vi "keccak.core.vi"(10 "keccak.i":u16, 11 "state[24]":u64[](array[numeric])=[0, 0, 0, 0, 0, 0, 0, 0, 0, 0, 0, 0, 0, 0, 0, 0, 0, 0, 0, 0, 0, 0, 0, 0] format="%.0x") -> (3 "Ebx":u64[](array[numeric]) format="%.0x")   [LabVIEW 2021]
uses:
  host.impl/Step.4.5.6.7.Inputs.ctl
panel:
  out "New.State":u64[](array[numeric])
  out "Exy":u64[](array[numeric]) format="%.0x"
  out "Step.8.Dx":u64[](array[numeric]) format="%.0x"
  out "state[24].out":u64[](array[numeric]) format="%.0x"
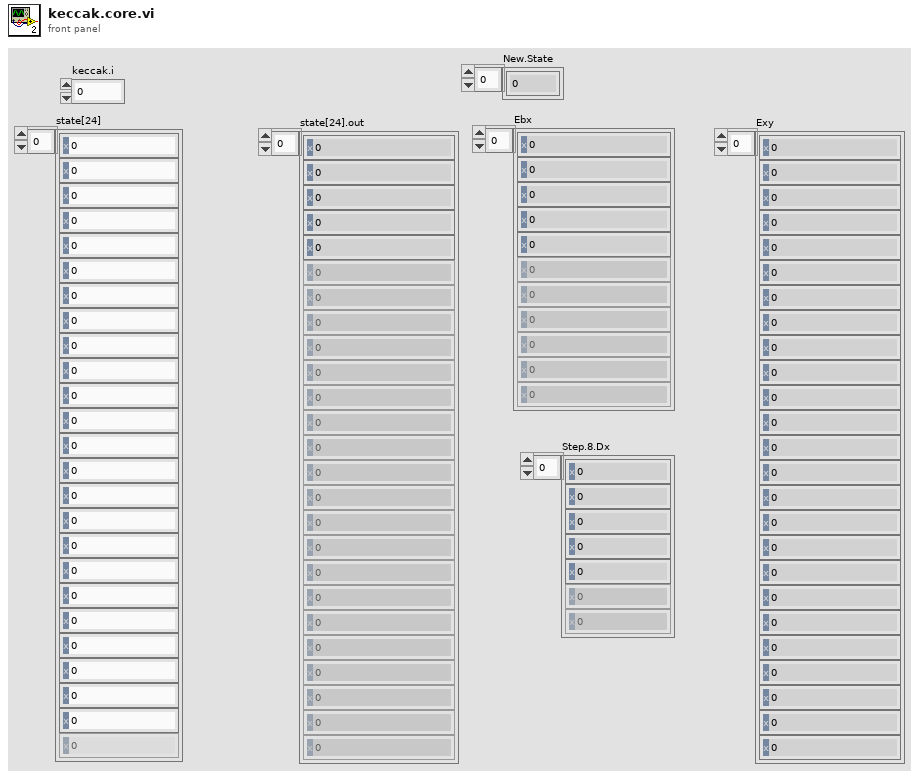
[diagram p1: front panel]
types:
  T1 = typedef "Step.4.5.6.7.Inputs.ctl" = cluster{"Left_Shift":i32, "State_Index":i32, "D_Index":i32}
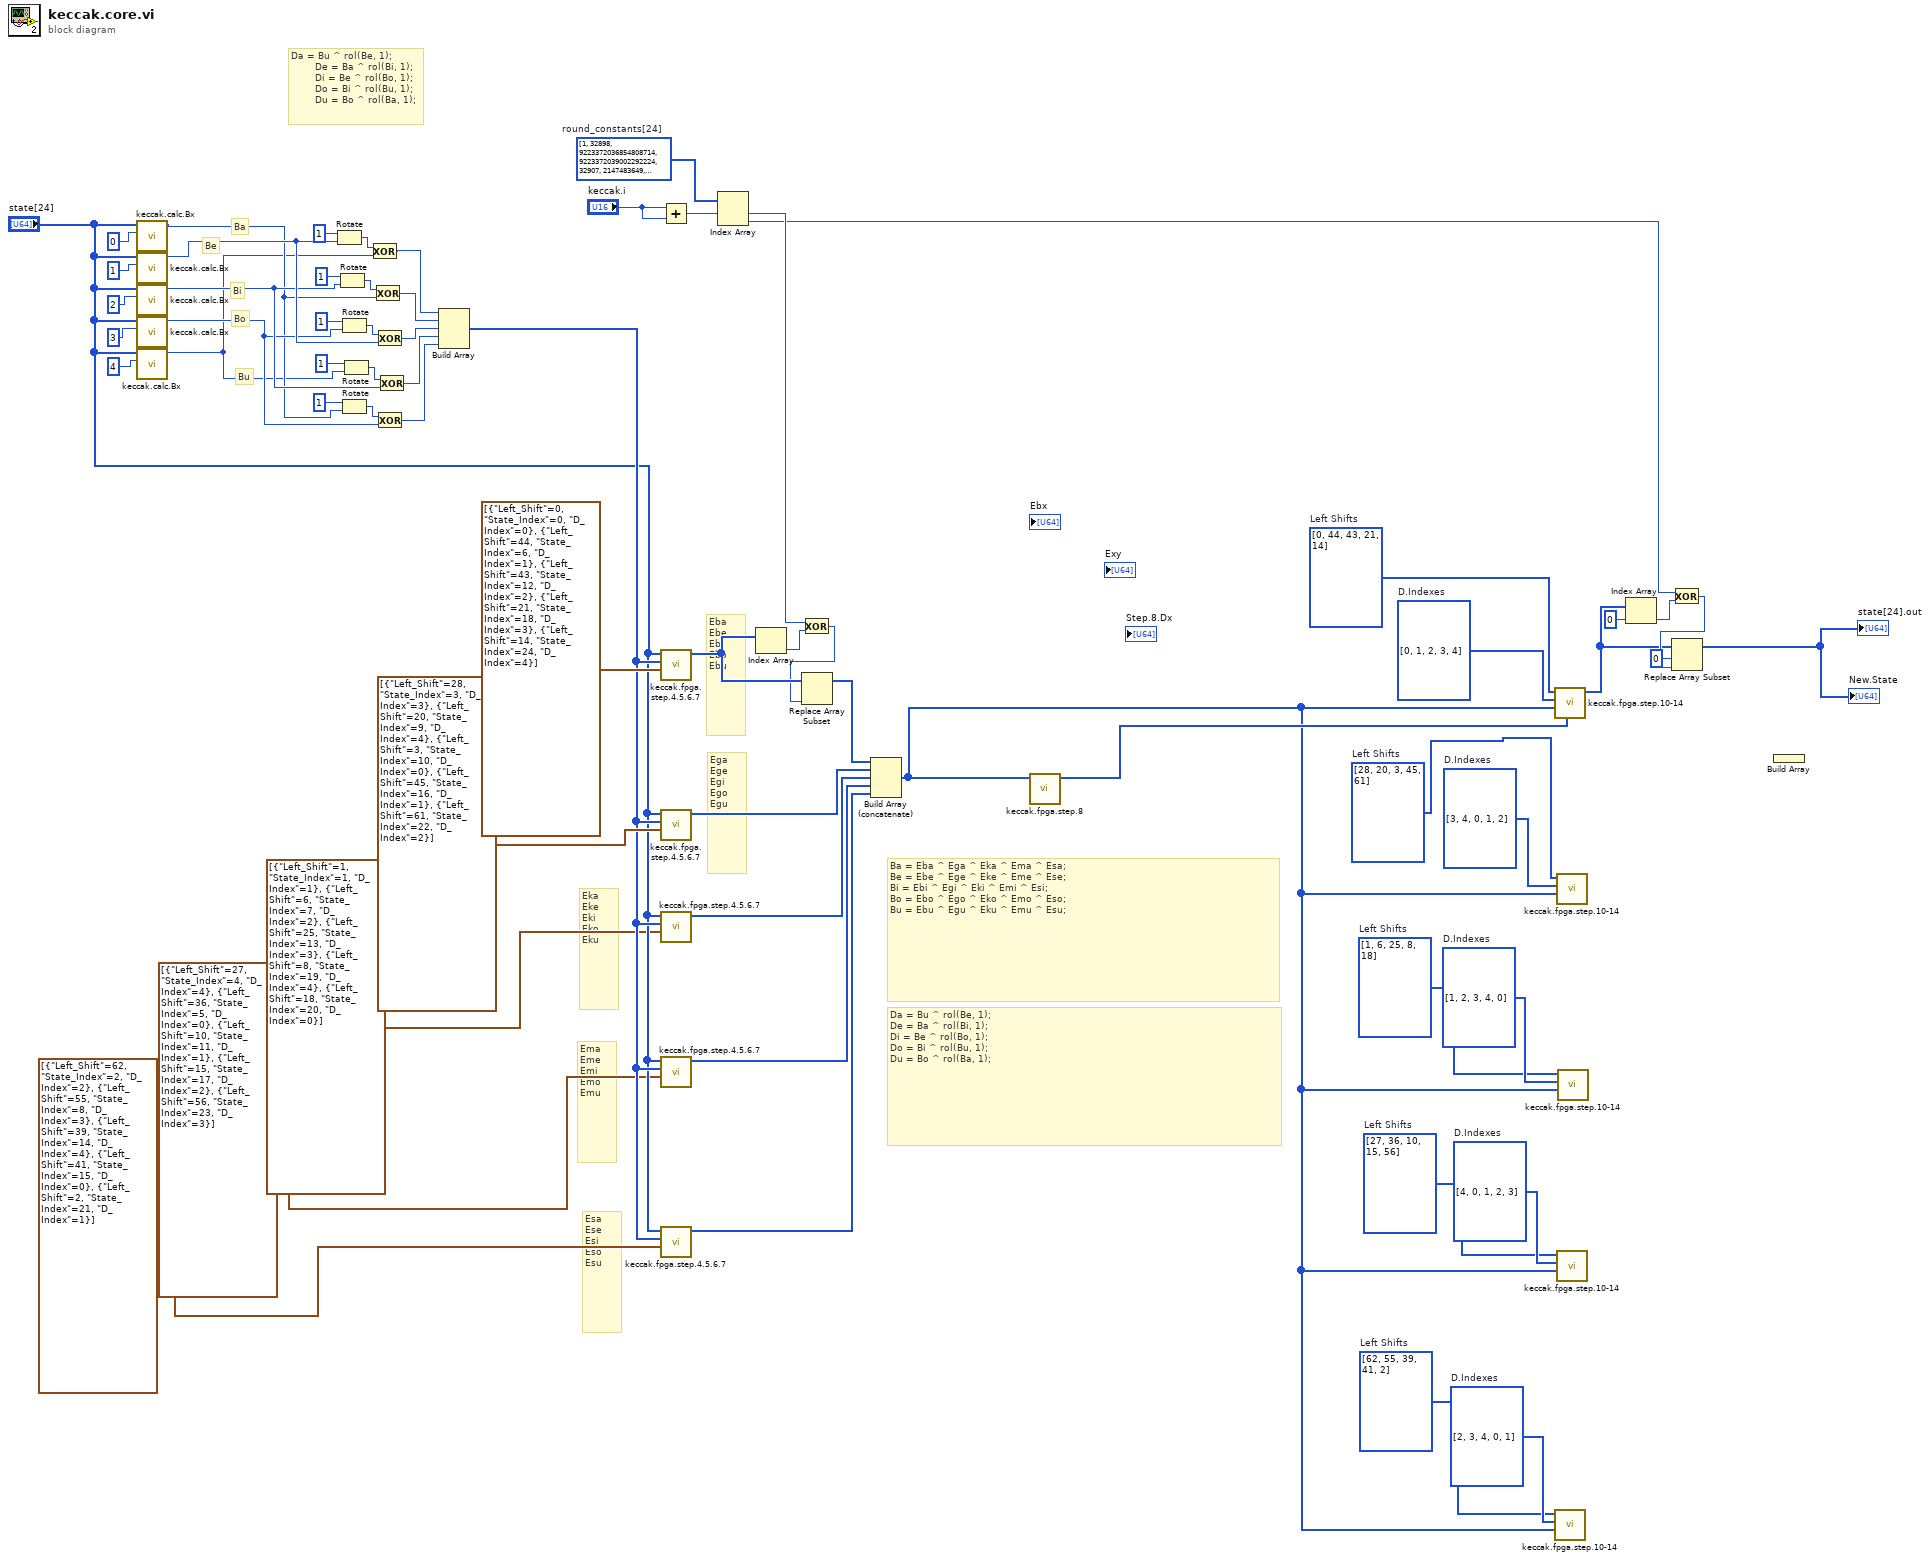
[diagram p0: block diagram]
diagram:
  w5 = i32[] [2, 3, 4, 0, 1]  # D.Indexes
  w6 = i32[] [4, 0, 1, 2, 3]  # D.Indexes
  w7 = i32[] [1, 2, 3, 4, 0]  # D.Indexes
  w8 = i32[] [3, 4, 0, 1, 2]  # D.Indexes
  w1 = i32[] [62, 55, 39, 41, 2]  # Left Shifts
  w2 = i32[] [27, 36, 10, 15, 56]  # Left Shifts
  w3 = i32[] [1, 6, 25, 8, 18]  # Left Shifts
  w4 = i32[] [28, 20, 3, 45, 61]  # Left Shifts
  w17 = i32[] [0, 1, 2, 3, 4]  # D.Indexes
  w18 = i32[] [0, 44, 43, 21, 14]  # Left Shifts
  w36 = u64[] [1, 32898, 9223372036854808714, 9223372039002292224, 32907, 2147483649, 9223372039002292353, 9223372036854808585, 138, 136, 2147516425, 2147483658, 2147516555, 9223372036854775947, 9223372036854808713, 9223372036854808579, 9223372036854808578, 9223372036854775936, 32778, 9223372039002259466, 9223372039002292353, 9223372036854808704, 2147483649, 9223372039002292232]  # round_constants[24]
  # "Da = Bu ^ rol(Be, 1);\nDe = Ba ^ rol(Bi, 1);\nDi = Be ^ rol(Bo, 1);\nDo = Bi ^ rol(Bu, 1);\nDu = Bo ^ rol(Ba, 1);"
  # "Ba = Eba ^ Ega ^ Eka ^ Ema ^ Esa;\nBe = Ebe ^ Ege ^ Eke ^ Eme ^ Ese;\nBi = Ebi ^ Egi ^ Eki ^ Emi ^ Esi;\nBo = Ebo ^ Ego ^ Eko ^ Emo ^ Eso;\nBu = Ebu ^ Egu ^ Eku ^ Emu ^ Esu;"
  # "Esa\nEse\nEsi\nEso\nEsu"
  # "Ema\nEme\nEmi\nEmo\nEmu"
  # "Eka\nEke\nEki\nEko\nEku"
  # "Ega\nEge\nEgi\nEgo\nEgu"
  # "Eba\nEbe\nEbi\nEbo\nEbu"
  # "Bu"
  # "Bo"
  # "Bi"
  # "Be"
  # "Ba"
  # "Da = Bu ^ rol(Be, 1);\n        De = Ba ^ rol(Bi, 1);\n        Di = Be ^ rol(Bo, 1);\n        Do = Bi ^ rol(Bu, 1);\n        Du = Bo ^ rol(Ba, 1);"
  n1 = call "keccak.calc.Bx.vi"("index"=0, "state[24]"="state[24]") -> ("Numeric"=w60:u64)  [unwired: 9 in]
  n2 = call "keccak.calc.Bx.vi"("index"=1, "state[24]"="state[24]") -> ("Numeric"=w63:u64)  [unwired: 9 in]
  n3 = call "keccak.calc.Bx.vi"("index"=2, "state[24]"="state[24]") -> ("Numeric"=w62:u64)  [unwired: 9 in]
  n4 = call "keccak.calc.Bx.vi"("index"=3, "state[24]"="state[24]") -> ("Numeric"=w61:u64)  [unwired: 9 in]
  n5 = call "keccak.calc.Bx.vi"("index"=4, "state[24]"="state[24]") -> ("Numeric"=w57:u64)  [unwired: 9 in]
  n6 = Rotate(1:w63, 2:i16 1 ("y")) -> (0:w50:u64)
  n7 = Rotate(1:w62, 2:i16 1 ("y")) -> (0:w52:u64)
  n8 = Rotate(1:w61, 2:i16 1 ("y")) -> (0:w54:u64)
  n9 = Rotate(1:w60, 2:i16 1 ("y")) -> (0:w59:u64)
  n10 = Rotate(1:w57, 2:i16 1 ("y")) -> (0:w56:u64)
  n11 = Exclusive Or(1:w57, 2:w50) -> (0:w43:u64)
  n12 = Exclusive Or(1:w60, 2:w52) -> (0:w42:u64)
  n13 = Exclusive Or(1:w63, 2:w54) -> (0:w41:u64)
  n14 = Exclusive Or(1:w61, 2:w59) -> (0:w39:u64)
  n15 = Exclusive Or(1:w62, 2:w56) -> (0:w40:u64)
  n16 = Build Array(w43, w42, w41, w40, w39) -> (w29:u64[])
  n17 = Add(x="keccak.i", y="keccak.i") -> (x+y=w35:u16)
  n18 = call "keccak.fpga.step.4.5.6.7.vi"("E.Parameters"=T1[] [{"Left_Shift"=0, "State_Index"=0, "D_Index"=0}, {"Left_Shift"=44, "State_Index"=6, "D_Index"=1}, {"Left_Shift"=43, "State_Index"=12, "D_Index"=2}, {"Left_Shift"=21, "State_Index"=18, "D_Index"=3}, {"Left_Shift"=14, "State_Index"=24, "D_Index"=4}], "D.in"=w29, "state[24]"="state[24]") -> ("Exy.out"=w33:u64[])  [unwired: 8 in]
  n19 = call "keccak.fpga.step.4.5.6.7.vi"("E.Parameters"=T1[] [{"Left_Shift"=28, "State_Index"=3, "D_Index"=3}, {"Left_Shift"=20, "State_Index"=9, "D_Index"=4}, {"Left_Shift"=3, "State_Index"=10, "D_Index"=0}, {"Left_Shift"=45, "State_Index"=16, "D_Index"=1}, {"Left_Shift"=61, "State_Index"=22, "D_Index"=2}], "D.in"=w29, "state[24]"="state[24]") -> ("Exy.out"=w24:u64[])  [unwired: 8 in]
  n20 = call "keccak.fpga.step.4.5.6.7.vi"("E.Parameters"=T1[] [{"Left_Shift"=1, "State_Index"=1, "D_Index"=1}, {"Left_Shift"=6, "State_Index"=7, "D_Index"=2}, {"Left_Shift"=25, "State_Index"=13, "D_Index"=3}, {"Left_Shift"=8, "State_Index"=19, "D_Index"=4}, {"Left_Shift"=18, "State_Index"=20, "D_Index"=0}], "D.in"=w29, "state[24]"="state[24]") -> ("Exy.out"=w23:u64[])  [unwired: 8 in]
  n21 = call "keccak.fpga.step.4.5.6.7.vi"("E.Parameters"=T1[] [{"Left_Shift"=27, "State_Index"=4, "D_Index"=4}, {"Left_Shift"=36, "State_Index"=5, "D_Index"=0}, {"Left_Shift"=10, "State_Index"=11, "D_Index"=1}, {"Left_Shift"=15, "State_Index"=17, "D_Index"=2}, {"Left_Shift"=56, "State_Index"=23, "D_Index"=3}], "D.in"=w29, "state[24]"="state[24]") -> ("Exy.out"=w22:u64[])  [unwired: 8 in]
  n22 = call "keccak.fpga.step.4.5.6.7.vi"("E.Parameters"=T1[] [{"Left_Shift"=62, "State_Index"=2, "D_Index"=2}, {"Left_Shift"=55, "State_Index"=8, "D_Index"=3}, {"Left_Shift"=39, "State_Index"=14, "D_Index"=4}, {"Left_Shift"=41, "State_Index"=15, "D_Index"=0}, {"Left_Shift"=2, "State_Index"=21, "D_Index"=1}], "D.in"=w29, "state[24]"="state[24]") -> ("Exy.out"=w21:u64[])  [unwired: 8 in]
  n23 = Index Array(array=w36, index #1=w35) -> (element #1=w31:u64, element #2=w11:u64)  [unwired: 1 in]
  n24 = Index Array(array=w33) -> (element=w34:u64)  [unwired: 1 in]
  n25 = Exclusive Or(1:w34, 2:w31) -> (0:w32:u64)
  n26 = Replace Array Subset(array=w33, new element=w32) -> (w20:u64[])  [unwired: 1 in]
  n27 = Build Array (concatenate)(w20, w24, w23, w22, w21) -> (w9:u64[])
  n28 = call "keccak.fpga.step.8.vi"("Exy.in"=w9) -> ("Step.8.Dx"=w19:u64[])  [unwired: 10 in]
  n29 = call "keccak.fpga.step.10-14.vi"("Step.8.Dx"=w19, "Exy.in"=w9, "D.Indexes"=w17, "Left Shifts"=w18) -> ("New.State"=w12:u64[])  [unwired: 7 in]
  n30 = call "keccak.fpga.step.10-14.vi"("Exy.in"=w9, "D.Indexes"=w5, "Left Shifts"=w1) -> ()  [unwired: 8 in, 1 out]
  n31 = call "keccak.fpga.step.10-14.vi"("Exy.in"=w9, "D.Indexes"=w8, "Left Shifts"=w4) -> ()  [unwired: 8 in, 1 out]
  n32 = call "keccak.fpga.step.10-14.vi"("Exy.in"=w9, "D.Indexes"=w6, "Left Shifts"=w2) -> ()  [unwired: 8 in, 1 out]
  n33 = call "keccak.fpga.step.10-14.vi"("Exy.in"=w9, "D.Indexes"=w7, "Left Shifts"=w3) -> ()  [unwired: 8 in, 1 out]
  n34 = Index Array(array=w12, index=0) -> (element=w16:u64)
  n35 = Exclusive Or(1:w16, 2:w11) -> (0:w15:u64)
  n36 = Replace Array Subset(array=w12, new element=w15, index=0) -> (→"state[24].out" →"New.State":u64[])
  n37 = Build Array() -> ()  [unwired: 1 in, 1 out]
